vi "Tip Shaper.vi"() -> ()   [LabVIEW 2016]
doc: "Performs a configurable bias/Z sequence that can help to shape a STM tip.\n\n- Nanonis Programming Interface -"
uses:
  Nanonis Prog Interface.lvlib
panel:
  in  "Current Gain":u16(ring) items=["HS 10^5", "HS 10^6", "HS 10^7", "HS 10^8", "HS 10^9", "HS 10^10", "HS 10^11", "LN 10^3", "LN 10^4", "LN 10^5", "LN 10^6", "LN 10^7", "LN 10^8", "LN 10^9"]
  in  "Bias value":dbl=1.0 format="%.3p"
  in  "Change Bias":bool=TRUE
  in  "Switch Gain":bool=TRUE
  in  "Draw":bool=TRUE
  in  "Lift Time 1":dbl=0.2 min=0.02 max=600.0 format="%.2p"
  out "Bias (V)":sgl format="%_5p"
  in  "Feedback":bool=TRUE
  out "oStartSequence":refnum<k4>
  in  "cleanTip":bool
  out "allQuit":bool
  in  "quit":bool
  out "oUpdateDisplay":refnum<k4>
  in  "End Wait Time":dbl=0.1 format="%.2p"
  in  "Lifting Bias":dbl=2.0 format="%.3p"
  in  "Lift Time 2":dbl=1.0 min=0.02 max=600.0 format="%.2p"
  in  "Lift Height":dbl=5e-09 format="%.2p"
  in  "Switch Off Delay":dbl=0.10999999999999999 format="%.2p"
  in  "Bias Settling Time":dbl=0.09999999999999999 format="%.2p"
  in  "TipLift":dbl=-2e-10 format="%.2p"
  out "Z Graph":cluster{dbl[], dbl[]}[](graph)=[{[0.0, 0.10999999999999999, 0.10999999999999999, 0.20999999999999996, 0.41, 0.41, 0.51, 1.51, 1.51, 1.61], [0.0, 0.0, 0.0, 0.0, -2e-10, -2e-10, -2e-10, 5e-09, 5e-09, 5e-09]}, {[0.0, 0.10999999999999999, 0.10999999999999999, 0.20999999999999996, 0.41, 0.41, 0.51, 1.51, 1.51, 1.61], [0.0, 0.0, 1.0, 1.0, 1.0, 2.0, 2.0, 2.0, 0.0, 0.0]}]
  # "Parameters"
  # "Internal Variables"
  # "s"
  # "V"
  # "m"
  # "s"
  # "V"
  # "s"
  # "m"
  # "s"
  # "s"
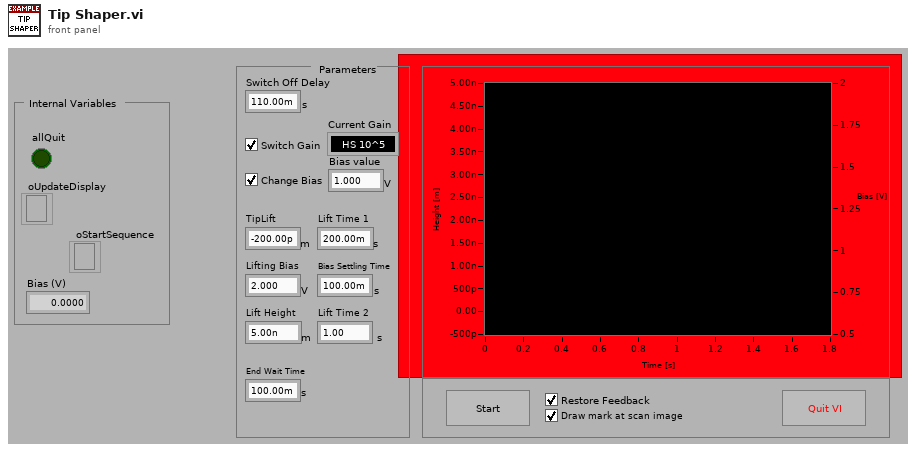
[diagram p1: front panel]
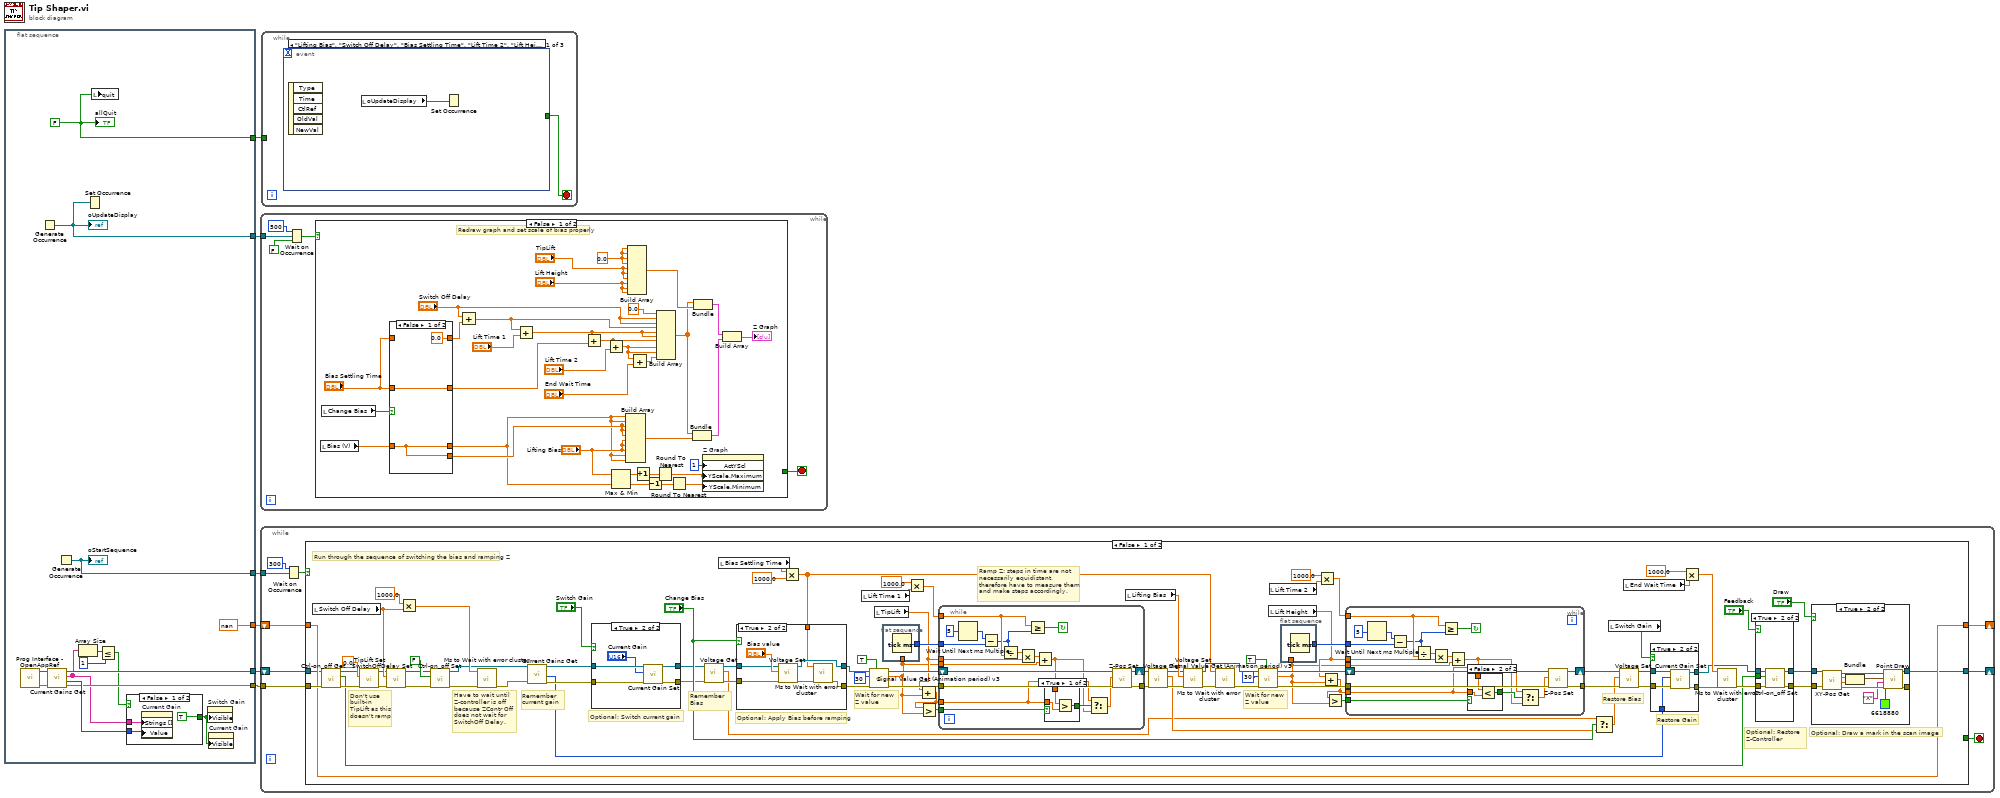
[diagram p0: block diagram]
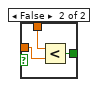
[diagram p6: hidden frame]
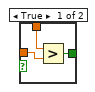
[diagram p8: hidden frame]
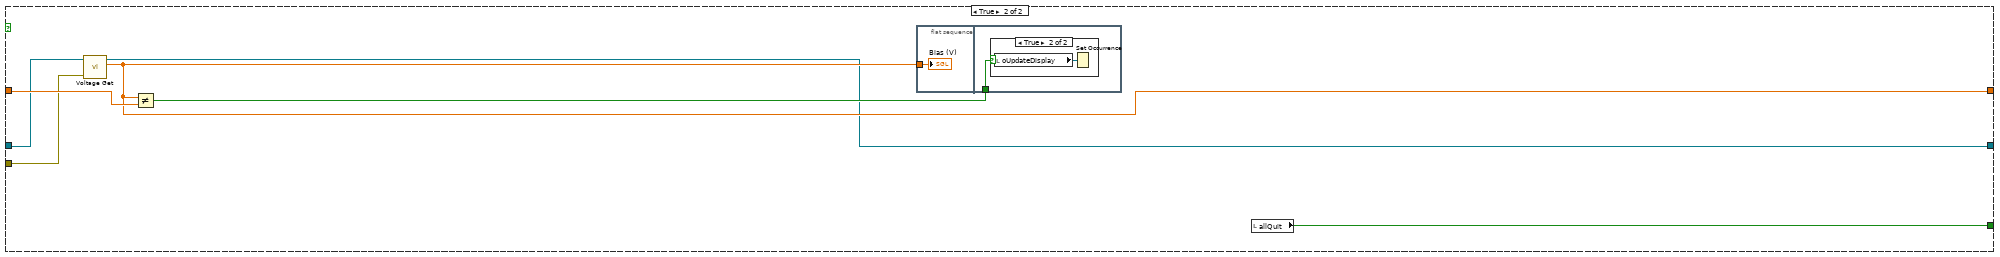
[diagram p9: hidden frame]
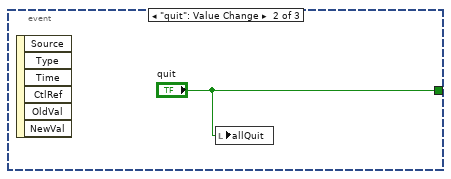
[diagram p11: hidden frame]
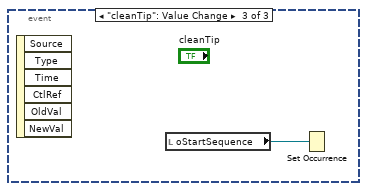
[diagram p12: hidden frame]
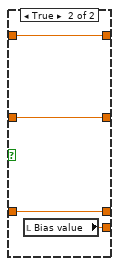
[diagram p13: hidden frame]
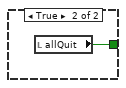
[diagram p14: hidden frame]
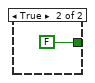
[diagram p15: hidden frame]
diagram:
  n1 = flat-sequence {
    tunnel: [w18] -> w6
    tunnel: [w20] -> w5
    tunnel: [w19] -> w4
    tunnel: [w12] -> w3
    tunnel: [sgl nan ("Bias (V)")] -> w2
    tunnel: [w13] -> w1
    frame #0 {
      w18 = FALSE ("allQuit")
      n2 = call <userlib>:"Prog Interface - OpenAppRef.vi"() -> ("Error out"=w14:errorcluster, "Application reference"=w15:refnum<vi>)  [unwired: 6 in]
      n3 = Generate Occurrence() -> (w20:refnum<k4>)
      "oUpdateDisplay" <- w20
      n4 = call <userlib>:"Current Gains Get.vi"("Error in (no error)"=w14, "Application ref in"=w15) -> ("Error out"=w12:errorcluster, "Selected Gain"=w16:u16, "Gains"=w11:string[], "Application ref out"=w13:refnum<vi>)  [unwired: 6 in]
      n5 = Generate Occurrence() -> (w19:refnum<k4>)
      "oStartSequence" <- w19
      n6 = Array Size(array=w11) -> (size(s)=w10:i32)
      n7 = Set Occurrence(w20) -> ()
      n8 = local write "quit"(w18) -> ()
      n9 = Less Or Equal?(x=w10, y=1) -> (x <= y?=w8:bool)
      n10 = case shown="False" w8 {
        tunnel: w16 -> [w23 _]
        tunnel: w11 -> [w22 _]
        tunnel: [TRUE FALSE] -> w7
        frame False {
          n11 = property on="Current Gain" class="Ring (strict)"("Strings []"=w22, "Value"=w23) -> ()  [unwired: 2 in, 2 out]
        }
        frame True {
        }
      }
      n12 = property on="Switch Gain" class="Bool (strict)"("Visible"=w7) -> ()  [unwired: 2 in, 2 out]
      n13 = property on="Current Gain" class="Ring (strict)"("Visible"=w7) -> ()  [unwired: 2 in, 2 out]
      "allQuit" <- w18
    }
  }
  n14 = while {
    tunnel: w5 -> [w25]
    stop <- w28 stop-if-true
    n15 = Wait on Occurrence(1:FALSE ("ignore previous (T)"), 2:w25, 3:500 ("ms timeout (-1)")) -> (0:w29:bool)
    n16 = case shown="False" w29 {
      tunnel: [_ w71] -> w28
      frame False {
        w39 = 0.0 ("new element/subarray")
        # "Redraw graph and set scale of bias properly"
        n17 = local read "Bias (V)"() -> (w33:sgl)
        n18 = local read "Change Bias"() -> (w32:bool)
        n19 = case shown="False" w32 {
          tunnel: [0.0 ("Bias Settling Time (s)") w70] -> w36
          tunnel: "Bias Settling Time" -> [_ w70]
          tunnel: [w64 w67] -> w31
          tunnel: [w66 w69] -> w35
          tunnel: "Bias Settling Time" -> [w66 w69]
          tunnel: [w64 w68] -> w30
          tunnel: w33 -> [w64 w68]
          frame False {
          }
          frame True {
            n20 = local read "Bias value"() -> (w67:dbl)
          }
        }
        n21 = Add(x="Switch Off Delay", y=w36) -> (x+y=w37:dbl)
        n22 = Add(x=w37, y="Lift Time 1") -> (x+y=w41:dbl)
        n23 = Add(x=w41, y=w35) -> (x+y=w42:dbl)
        n24 = Add(x=w42, y="Lift Time 2") -> (x+y=w60:dbl)
        n25 = Max & Min(x="Lifting Bias", y=w30) -> (max(x,y)=w48:dbl, min(x,y)=w47:dbl)
        n26 = Build Array(w30, w30, w31, w31, w31, "Lifting Bias", "Lifting Bias", "Lifting Bias", w30, w30) -> (w52:dbl[])
        n27 = Build Array(w39, w39, w39, w39, "TipLift", "TipLift", "TipLift", "Lift Height", "Lift Height", "Lift Height") -> (w57:dbl[])
        n28 = Add(x=w60, y="End Wait Time") -> (x+y=w59:dbl)
        n29 = Increment(x=w48) -> (x+1=w49:dbl)
        n30 = Decrement(x=w47) -> (x-1=w46:dbl)
        n31 = Round To Nearest(number=w49) -> (nearest integer value=w50:dbl)
        n32 = Build Array(0.0 ("new element/subarray"), "Switch Off Delay", "Switch Off Delay", w37, w41, w41, w42, w60, w60, w59) -> (w53:dbl[])
        n33 = Round To Nearest(number=w46) -> (nearest integer value=w51:dbl)
        n34 = Bundle(w53, w52) -> (w55:cluster{dbl[], dbl[]})  [unwired: 1 in]
        n35 = Bundle(w53, w57) -> (w56:cluster{dbl[], dbl[]})  [unwired: 1 in]
        n36 = property on="Z Graph" class="XYGraph (strict)"("ActYScl"=1 ("Active Y Scale"), "YScale.Maximum"=w50, "YScale.Minimum"=w51) -> ()  [unwired: 2 in, 2 out]
        n37 = Build Array(w56, w55) -> (→"Z Graph":cluster{dbl[], dbl[]}[])
      }
      frame True {
        n38 = local read "allQuit"() -> (w71:bool)
      }
    }
  }
  n39 = while {
    tunnel: w4 -> [w78]
    tunnel: w3 -> [w76]
    shift-right: [w74] -> _
    shift-left: w2 -> [w75]
    shift-right: [w72] -> _
    shift-left: w1 -> [w73]
    stop <- w77 stop-if-true
    n40 = Wait on Occurrence(2:w78, 3:300 ("ms timeout (-1)")) -> (0:w79:bool)  [unwired: 1 in]
    n41 = case shown="False" w79 {
      tunnel: [_ w264] -> w77
      tunnel: w76 -> [w144 w260]
      tunnel: w75 -> [w141 w262]
      tunnel: [w141 w261] -> w74
      tunnel: w73 -> [w126 w259]
      tunnel: [w111 w258] -> w72
      frame False {
        # "Ramp Z: steps in time are not necessarily equidistant, therefore have to measure them and make steps accordingly."
        # "Optional: Draw a mark in the scan image"
        # "Optional: Apply Bias before ramping"
        # "Remember Bias"
        # "Optional: Switch current gain"
        # "Remember current gain"
        # "Restore Bias"
        # "Optional: Restore Z-Controller"
        # "Restore Gain"
        # "Don't use built-in TipLift as this doesn't ramp"
        # "Wait for new Z value"
        # "Have to wait until Z-controller is off because ZContr Off does not wait for SwitchOff Delay."
        # "Wait for new Z value"
        # "Run through the sequence of switching the bias and ramping Z"
        n42 = local read "Switch Off Delay"() -> (w152:dbl)
        n43 = call <userlib>:"Ctrl-on_off Get.vi"("error in (no error)"=w144, "Application ref in"=w126) -> ("error out"=w143:errorcluster, "Z-Controller on/off status"=w142:bool, "Application ref out"=w125:refnum<vi>)  [unwired: 7 in]
        n44 = call <userlib>:"TipLift Set.vi"("error in (no error)"=w143, "TipLift (m)"=sgl 0.0, "Application ref in"=w125) -> ("error out"=w163:errorcluster, "Application ref out"=w124:refnum<vi>)  [unwired: 7 in]
        n45 = call <userlib>:"SwitchOffDelay Set.vi"("error in (no error)"=w163, "Switch off Delay (s)"=w152, "Application ref in"=w124) -> ("error out"=w132:errorcluster, "Application ref out"=w123:refnum<vi>)  [unwired: 7 in]
        n46 = Multiply(x=1000.0, y=w152) -> (x*y=w140:dbl)
        n47 = call <userlib>:"Ctrl-on_off Set.vi"("error in (no error)"=w132, "Z Controller ON/OFF"=FALSE, "Application ref in"=w123) -> ("error out"=w148:errorcluster, "Application ref out"=w98:refnum<vi>)  [unwired: 7 in]
        n48 = call "Ms to Wait with error cluster.vi"("error in (no error)"=w148, "milliseconds to wait"=w140) -> ("error out"=w96:errorcluster)  [unwired: 4 in, 1 out]
        n49 = call <userlib>:"Current Gains Get.vi"("Error in (no error)"=w96, "Application ref in"=w98) -> ("Error out"=w95:errorcluster, "Selected Gain"=w89:u16, "Application ref out"=w97:refnum<vi>)  [unwired: 6 in, 1 out]
        n50 = case shown="True" "Switch Gain" {
          tunnel: w97 -> [w181 w186]
          tunnel: w95 -> [w180 w185]
          tunnel: [w181 w183] -> w103
          tunnel: [w180 w184] -> w101
          frame False {
          }
          frame True {
            n51 = call <userlib>:"Current Gain Set.vi"("Error in (no error)"=w185, "Gain index"="Current Gain", "Application ref in"=w186) -> ("Error out"=w184:errorcluster, "Application ref out"=w183:refnum<vi>)  [unwired: 7 in]
          }
        }
        n52 = call <userlib>:"Voltage Get.vi"("error in (no error)"=w101, "Application ref in"=w103) -> ("error out"=w100:errorcluster, "Bias (V)"=w99:sgl, "Application ref out"=w102:refnum<vi>)  [unwired: 7 in]
        n53 = local read "Bias Settling Time"() -> (w150:dbl)
        n54 = Multiply(x=w150, y=1000.0) -> (x*y=w107:dbl)
        n55 = case shown="True" "Change Bias" {
          tunnel: w102 -> [w172 w174]
          tunnel: [w172 w178] -> w109
          tunnel: w100 -> [w171 w173]
          tunnel: [w171 w177] -> w108
          tunnel: w107 -> [_ w176]
          frame False {
          }
          frame True {
            n56 = call <userlib>:"Voltage Set.vi"("Error in (no error)"=w173, "Bias (V)"="Bias value", "Application ref in"=w174) -> ("Error out"=w179:errorcluster, "Application ref out"=w178:refnum<vi>)  [unwired: 7 in]
            n57 = call "Ms to Wait with error cluster.vi"("error in (no error)"=w179, "milliseconds to wait"=w176) -> ("error out"=w177:errorcluster)  [unwired: 4 in, 1 out]
          }
        }
        n58 = local read "Lift Time 1"() -> (w130:dbl)
        n59 = call <userlib>:"Signal Value Get (Animation period) v3.vi"("Wait for newest data (F=False)"=TRUE ("Wait for newest data (F)"), "error in (no error)"=w108, "Signal index (0-127)"=i8 30 ("Signal index (0-23)"), "Application ref in"=w109) -> ("error out"=w135:errorcluster, "Signal value"=w86:sgl, "Application ref out"=w121:refnum<vi>)  [unwired: 4 in]
        n60 = local read "TipLift"() -> (w88:dbl)
        n61 = flat-sequence {
          tunnel: [w199] -> w134
          tunnel: w86 -> [_]
          frame #0 {
            n62 = Tick Count (ms)() -> (millisecond timer value=w199:u32)
          }
        }
        n63 = Multiply(x=1000.0, y=w130) -> (x*y=w129:dbl)
        n64 = Add(x=w88, y=w86) -> (x+y=w87:dbl)
        n65 = Greater?(x=w87, y=w86) -> (0:w85:bool)
        n66 = while {
          tunnel: w134 -> [w218]
          tunnel: w88 -> [w216]
          tunnel: [w215] -> w128
          tunnel: w86 -> [w211]
          tunnel: w135 -> [w212]
          tunnel: w129 -> [w209]
          shift-right: [w205] -> w120
          shift-left: w121 -> [w206]
          tunnel: w87 -> [w202]
          tunnel: w85 -> [w204]
          stop <- w217 continue-if-true
          n67 = Wait Until Next ms Multiple(millisecond multiple=u32 5) -> (millisecond timer value=w208:u32)
          n68 = Subtract(x=w208, y=w218) -> (x-y=w207:u32)
          n69 = Divide(x=w207, y=w209) -> (x/y=w213:dbl)
          n70 = Multiply(x=w213, y=w216) -> (x*y=w210:dbl)
          n71 = Greater Or Equal?(x=w209, y=w207) -> (x >= y?=w217:bool)
          n72 = Add(x=w210, y=w211) -> (x+y=w201:dbl)
          n73 = case shown="True" w204 {
            tunnel: w201 -> [w221 w224]
            tunnel: w202 -> [w220 w223]
            tunnel: [w219 w222] -> w203
            frame True {
              n74 = Greater?(x=w221, y=w220) -> (0:w219:bool)
            }
            frame False {
              n75 = Less?(x=w224, y=w223) -> (x < y?=w222:bool)
            }
          }
          n76 = Select(t=w202, s=w203, f=w201) -> (s? t:f=w200:dbl)
          n77 = call <userlib>:"Z-Pos Set.vi"("error in (no error)"=w212, "Z position (m)"=w200, "Application ref in"=w206) -> ("error out"=w215:errorcluster, "Application ref out"=w205:refnum<vi>)  [unwired: 7 in]
        }
        n78 = local read "Lifting Bias"() -> (w162:dbl)
        n79 = call <userlib>:"Voltage Get.vi"("error in (no error)"=w128, "Application ref in"=w120) -> ("error out"=w127:errorcluster, "Bias (V)"=w105:sgl, "Application ref out"=w119:refnum<vi>)  [unwired: 7 in]
        n80 = call <userlib>:"Voltage Set.vi"("Error in (no error)"=w127, "Bias (V)"=w162, "Application ref in"=w119) -> ("Error out"=w147:errorcluster, "Application ref out"=w115:refnum<vi>)  [unwired: 7 in]
        n81 = call "Ms to Wait with error cluster.vi"("error in (no error)"=w147, "milliseconds to wait"=w107) -> ("error out"=w139:errorcluster)  [unwired: 4 in, 1 out]
        n82 = call <userlib>:"Signal Value Get (Animation period) v3.vi"("Wait for newest data (F=False)"=TRUE ("Wait for newest data (F)"), "error in (no error)"=w139, "Signal index (0-127)"=i8 30 ("Signal index (0-23)"), "Application ref in"=w115) -> ("error out"=w138:errorcluster, "Signal value"=w83:sgl, "Application ref out"=w117:refnum<vi>)  [unwired: 4 in]
        n83 = local read "Lift Height"() -> (w84:dbl)
        n84 = local read "Lift Time 2"() -> (w160:dbl)
        n85 = flat-sequence {
          tunnel: [w225] -> w156
          tunnel: w83 -> [_]
          frame #0 {
            n86 = Tick Count (ms)() -> (millisecond timer value=w225:u32)
          }
        }
        n87 = Multiply(x=1000.0, y=w160) -> (x*y=w149:dbl)
        n88 = Add(x=w84, y=w83) -> (x+y=w81:dbl)
        n89 = Greater?(x=w81, y=w83) -> (0:w82:bool)
        n90 = while {
          tunnel: w156 -> [w251]
          tunnel: w84 -> [w249]
          tunnel: [w248] -> w158
          tunnel: w83 -> [w244]
          tunnel: w138 -> [w245]
          tunnel: w149 -> [w242]
          shift-right: [w238] -> w116
          shift-left: w117 -> [w239]
          tunnel: w82 -> [w237]
          tunnel: w81 -> [w234]
          stop <- w250 continue-if-true
          n91 = Wait Until Next ms Multiple(millisecond multiple=u32 5) -> (millisecond timer value=w241:u32)
          n92 = Subtract(x=w241, y=w251) -> (x-y=w240:u32)
          n93 = Divide(x=w240, y=w242) -> (x/y=w246:dbl)
          n94 = Multiply(x=w246, y=w249) -> (x*y=w243:dbl)
          n95 = Greater Or Equal?(x=w242, y=w240) -> (x >= y?=w250:bool)
          n96 = Add(x=w243, y=w244) -> (x+y=w235:dbl)
          n97 = case shown="False" w237 {
            tunnel: w235 -> [w254 w257]
            tunnel: w234 -> [w253 w256]
            tunnel: [w252 w255] -> w236
            frame True {
              n98 = Greater?(x=w254, y=w253) -> (0:w252:bool)
            }
            frame False {
              n99 = Less?(x=w257, y=w256) -> (x < y?=w255:bool)
            }
          }
          n100 = Select(t=w234, s=w236, f=w235) -> (s? t:f=w233:dbl)
          n101 = call <userlib>:"Z-Pos Set.vi"("error in (no error)"=w245, "Z position (m)"=w233, "Application ref in"=w239) -> ("error out"=w248:errorcluster, "Application ref out"=w238:refnum<vi>)  [unwired: 7 in]
        }
        n102 = Select(t=w99, s="Change Bias", f=w105) -> (s? t:f=w104:sgl)
        n103 = local read "Switch Gain"() -> (w94:bool)
        n104 = call <userlib>:"Voltage Set.vi"("Error in (no error)"=w158, "Bias (V)"=w104, "Application ref in"=w116) -> ("Error out"=w91:errorcluster, "Application ref out"=w93:refnum<vi>)  [unwired: 7 in]
        n105 = local read "End Wait Time"() -> (w154:dbl)
        n106 = case shown="True" w94 {
          tunnel: w93 -> [w165 w170]
          tunnel: [w165 w169] -> w92
          tunnel: w91 -> [w164 w168]
          tunnel: [w164 w167] -> w90
          tunnel: w89 -> [_ w166]
          frame False {
          }
          frame True {
            n107 = call <userlib>:"Current Gain Set.vi"("Error in (no error)"=w168, "Gain index"=w166, "Application ref in"=w170) -> ("Error out"=w167:errorcluster, "Application ref out"=w169:refnum<vi>)  [unwired: 7 in]
          }
        }
        n108 = Multiply(x=1000.0, y=w154) -> (x*y=w145:dbl)
        n109 = call "Ms to Wait with error cluster.vi"("error in (no error)"=w90, "milliseconds to wait"=w145) -> ("error out"=w146:errorcluster)  [unwired: 4 in, 1 out]
        n110 = case shown="True" "Feedback" {
          tunnel: w146 -> [w226 w232]
          tunnel: w142 -> [_ w231]
          tunnel: w92 -> [w227 w230]
          tunnel: [w227 w229] -> w113
          tunnel: [w226 w228] -> w112
          frame False {
          }
          frame True {
            n111 = call <userlib>:"Ctrl-on_off Set.vi"("error in (no error)"=w232, "Z Controller ON/OFF"=w231, "Application ref in"=w230) -> ("error out"=w228:errorcluster, "Application ref out"=w229:refnum<vi>)  [unwired: 7 in]
          }
        }
        n112 = case shown="True" "Draw" {
          tunnel: w113 -> [w187 w198]
          tunnel: w112 -> [_ w196]
          tunnel: [w187 w194] -> w111
          tunnel: [_ w188] -> _
          frame False {
          }
          frame True {
            n113 = call <userlib>:"XY-Pos Get.vi"("error in (no error)"=w196, "Application ref in"=w198) -> ("error out"=w195:errorcluster, "Y (m)"=w192:sgl, "X (m)"=w193:sgl, "Application ref out"=w197:refnum<vi>)  [unwired: 5 in]
            n114 = Bundle("X (m)"=w193, "Y (m)"=w192) -> (w191:cluster{"X (m)":sgl, "Y (m)":sgl})  [unwired: 1 in]
            n115 = call <userlib>:"Point Draw.vi"("Application ref in"=w197, "Point Coordinates"=w191, "Text"="X", "Color"=u32 6618880, "error in (no error)"=w195) -> ("Application ref out"=w194:refnum<vi>, "error out"=w188:errorcluster)  [unwired: 9 in]
          }
        }
      }
      frame True {
        n116 = call <userlib>:"Voltage Get.vi"("error in (no error)"=w260, "Application ref in"=w259) -> ("Bias (V)"=w261:sgl, "Application ref out"=w258:refnum<vi>)  [unwired: 7 in, 1 out]
        n117 = Not Equal?(x=w261, y=w262) -> (x != y?=w263:bool)
        n118 = flat-sequence {
          tunnel: w261 -> [w265]
          tunnel: w263 -> [w266]
          frame #0 {
            "Bias (V)" <- w265
          }
          frame #1 {
            n119 = case shown="True" w266 {
              frame False {
              }
              frame True {
                n120 = local read "oUpdateDisplay"() -> (w267:refnum<k4>)
                n121 = Set Occurrence(w267) -> ()
              }
            }
          }
        }
        n122 = local read "allQuit"() -> (w264:bool)
      }
    }
  }
  n123 = while {
    tunnel: w6 -> [_]
    stop <- w268 stop-if-true
    n124 = event shown="[0] \"Lifting Bias\", \"Switch Off Delay\", \"Bias Settling Time\", \"Lift Time 2\", \"Lift Height\", \"End Wait Time\", \"TipLift\", \"Lift Time 1\", \"Change Bias\", \"Bias value\": Value Change" {
      selector: _ -> [_ _ _]
      dyn-events: _ -> [_ _ _]
      timeout: _ -> [_ _ _]
      tunnel: [_ "quit" _] -> w268
      event "Lifting Bias", "Switch Off Delay", "Bias Settling Time", "Lift Time 2", "Lift Height", "End Wait Time", "TipLift", "Lift Time 1", "Change Bias", "Bias value": Value Change {
        n125 = event-data() -> ()  [unwired: 1 in, 5 out]
        n126 = local read "oUpdateDisplay"() -> (w269:refnum<k4>)
        n127 = Set Occurrence(w269) -> ()
      }
      event "quit": Value Change {
        n128 = event-data() -> ()  [unwired: 1 in, 6 out]
        n129 = local write "allQuit"("quit") -> ()
      }
      event "cleanTip": Value Change {
        n130 = event-data() -> ()  [unwired: 1 in, 6 out]
        n131 = local read "oStartSequence"() -> (w271:refnum<k4>)
        n132 = Set Occurrence(w271) -> ()
      }
    }
  }
